vi "Func-Cp Cpk Calculation.vi"(0 "Uper limit":dbl=3.5, 5 "Lower limit":dbl=-3.5) -> (4 "Cp":dbl=1.932085875109604 format="%.3g", 6 "Cpk":dbl=1.7472929403358046 format="%.3g", 8 "Mean":dbl=-0.33475492991304356 format="%.3g", 10 "Variance":dbl=0.3646202027387419 format="%.3g", 15 "Standard deviation":dbl=0.6038378944209629 format="%.3g")   [LabVIEW 2015]
doc: "This Vi calculate the Cp and CPK of the population given by the Samples array.\nThe Upper and Lower limits need to be defined.\n\nCp= (UL-LL)/6*STD\n\nCpk= min((UL-MEAN)/3*STD,(MEAN-LL)/3*STD)"
panel:
  out "Data Length":dbl
  in  "문자열":string="-1.851121686\n-1.781249213\n-1.696262244\n-1.641406584\n-1.621321948\n-1.616843911\n-1.608642305\n-1.605459775\n-1.493903028\n-1.487135688\n-1.458574686\n-1.438584113\n-1.401760042\n-1.394260952\n-1.384378735\n-1.37466157\n-1.365849199\n-1.363884408\n-1.355128293\n-1.316161593\n-1.308444406\n-1.303143799\n-1.302773604\n-1.296959111\n-1.293790032\n-1.29178707\n-1.291699252\n-1.27635186\n-1.271757302\n-1.268175534\n-1.267821287\n-1.251471286\n-1.247559272\n-1.242962705\n-1.217645946\n-1.21736537\n-1.216009329\n-1.202190878\n-1.202112903\n-1.184886488\n-1.173962668\n-1.149552199\n-1.136492305\n-1.127663749\n-1.110186203\n-1.098839323\n-1.063263064\n-1.062590809\n-1.051174206\n-1.0350763\n-1.032616366\n-1.00586889\n-0.995767692\n-0.995159837\n-0.98525165\n-0.98196329\n-0.972898372\n-0.972202493\n-0.969240769\n-0.966011738\n-0.96122316\n-0.94254499\n-0.939456673\n-0.938051333\n-0.935893697\n-0.935341622\n-0.897347145\n-0.890632717\n-0.86677152\n-0.845623437\n-0.837863263\n-0.828699643\n-0.823162949\n-0.811628868\n-0.793890961\n-0.791592424\n-0.788485692\n-0.786059864\n-0.776439468\n-0.771175421\n-0.756713774\n-0.754180178\n-0.747972924\n-0.738974146\n-0.737735115\n-0.723125192\n-0.698505909\n-0.696495782\n-0.691014879\n-0.670102994\n-0.663213134\n-0.660173614\n-0.643176556\n-0.635550406\n-0.626554908\n-0.608300396\n-0.606095093\n-0.603400726\n-0.598510082\n-0.595354462\n-0.587561998\n-0.573913422\n-0.568345424\n-0.563687462\n-0.559160184\n-0.558902732\n-0.555301825\n-0.553530709\n-0.54605119\n-0.529988326\n-0.529235425\n-0.527026006\n-0.522869476\n-0.518973731\n-0.514763869\n-0.505587081\n-0.493579546\n-0.48985599\n-0.483537969\n-0.482482696\n-0.482414954\n-0.473320334\n-0.469467348\n-0.452348175\n-0.450832215\n-0.449496242\n-0.429675481\n-0.409118479\n-0.39707189\n-0.39029414\n-0.387083507\n-0.374743861\n-0.372941622\n-0.366007281\n-0.365920883\n-0.355394283\n-0.344413404\n-0.344094986\n-0.343650937\n-0.341575713\n-0.338731268\n-0.336521056\n-0.329717088\n-0.328186516\n-0.323740937\n-0.319114235\n-0.308047398\n-0.28295137\n-0.267773552\n-0.259518923\n-0.253211829\n-0.249036273\n-0.243012895\n-0.237937552\n-0.23472351\n-0.232765954\n-0.223881206\n-0.223762676\n-0.22323105\n-0.217884653\n-0.212155625\n-0.204602339\n-0.204030259\n-0.20356409\n-0.203086061\n-0.198433808\n-0.196635345\n-0.163945006\n-0.163916103\n-0.155360134\n-0.155235253\n-0.154121349\n-0.153919542\n-0.153388318\n-0.152636873\n-0.152481181\n-0.148134082\n-0.142589632\n-0.137008774\n-0.12647245\n-0.12557343\n-0.123881016\n-0.123868314\n-0.11561664\n-0.112112685\n-0.110043305\n-0.109985044\n-0.109723737\n-0.10594016\n-0.105639606\n-0.10355686\n-0.098659515\n-0.098607281\n-0.098373005\n-0.097118634\n-0.083297148\n-0.080455933\n-0.073766276\n-0.07251092\n-0.066247023\n-0.066247023\n-0.066045286\n-0.065259828\n-0.065034475\n-0.064515914\n-0.063829331\n-0.0599048\n-0.05223549\n-0.044948423\n-0.041152963\n-0.040847343\n-0.040683052\n-0.037970251\n-0.036130264\n-0.035842174\n-0.035620097\n-0.03546074\n-0.024837646\n-0.02259679\n-0.01924693\n-0.016197163\n-0.016091187\n-0.01588367\n-0.011912752\n-0.006533642\n-0.005783903\n-0.003741178\n-0.003713395\n-0.003698459\n-0.003577473\n0.006200636\n0.011377763\n0.015778103\n0.015778103\n0.016070206\n0.016334106\n0.028680123\n0.030356774\n0.03915029\n0.039653662\n0.05319111\n0.058159657\n0.059563761\n0.06034195\n0.060739363\n0.066268031\n0.067494866\n0.068603246\n0.06922644\n0.072871725\n0.07605783\n0.076936527\n0.079414977\n0.079762012\n0.081142904\n0.082046134\n0.083565072\n0.084937352\n0.08782068\n0.091087502\n0.099370535\n0.100358088\n0.108766379\n0.110649415\n0.137418853\n0.148535792\n0.16266193\n0.163330082\n0.169662436\n0.170493134\n0.222483436\n0.224152793\n0.230313209\n0.233322205\n0.234858871\n0.236222397\n0.237311582\n0.241024203\n0.258638946\n0.263582537\n0.282529822\n0.282695385\n0.286810418\n0.28940767\n0.296042548\n0.303273661\n0.304498374\n0.306697703\n0.306776635\n0.308335936\n0.323135697\n0.323585227\n0.330028997\n0.365758605\n0.386946878\n0.399114248\n0.409314606\n0.415204252\n0.431875391\n0.444799699\n0.466200899\n0.487349548\n0.491379186\n0.534357688\n0.536321157\n0.552104532\n0.553079385\n0.583193698\n0.600169278\n0.720360649\n0.722727719\n0.773414334\n0.827668935\n0.861770406\n0.868698608\n0.90552577\n1.02005817\n1.108558767\n1.130760164\n1.154642797\n1.223375919\n1.273115061"
  out "Samples":dbl[](array[numeric])=[-1.851121686, -1.781249213, -1.696262244, -1.641406584, -1.621321948, -1.616843911, -1.608642305, -1.605459775, -1.493903028, -1.487135688, -1.458574686, -1.438584113, -1.401760042, -1.394260952, -1.384378735, -1.37466157, -1.365849199, -1.363884408, -1.355128293, -1.316161593, -1.308444406, -1.303143799, -1.302773604, -1.296959111, -1.293790032, -1.29178707, -1.291699252, -1.27635186, -1.271757302, -1.268175534, -1.267821287, -1.251471286, -1.247559272, -1.242962705, -1.217645946, -1.21736537, -1.216009329, -1.202190878, -1.202112903, -1.184886488, -1.173962668, -1.149552199, -1.136492305, -1.127663749, -1.110186203, -1.098839323, -1.063263064, -1.062590809, -1.051174206, -1.0350763, -1.032616366, -1.00586889, -0.995767692, -0.995159837, -0.98525165, -0.98196329, -0.972898372, -0.972202493, -0.969240769, -0.966011738, -0.96122316, -0.94254499, -0.939456673, -0.938051333, -0.935893697, -0.935341622, -0.897347145, -0.890632717, -0.86677152, -0.845623437, -0.837863263, -0.828699643, -0.823162949, -0.811628868, -0.793890961, -0.791592424, -0.788485692, -0.786059864, -0.776439468, -0.771175421, -0.756713774, -0.754180178, -0.747972924, -0.738974146, -0.737735115, -0.723125192, -0.698505909, -0.696495782, -0.691014879, -0.670102994, -0.663213134, -0.660173614, -0.643176556, -0.635550406, -0.626554908, -0.608300396, -0.606095093, -0.603400726, -0.598510082, -0.595354462, -0.587561998, -0.573913422, -0.568345424, -0.563687462, -0.559160184, -0.558902732, -0.555301825, -0.553530709, -0.54605119, -0.529988326, -0.529235425, -0.527026006, -0.522869476, -0.518973731, -0.514763869, -0.505587081, -0.493579546, -0.48985599, -0.483537969, -0.482482696, -0.482414954, -0.473320334, -0.469467348, -0.452348175, -0.450832215, -0.449496242, -0.429675481, -0.409118479, -0.39707189, -0.39029414, -0.387083507, -0.374743861, -0.372941622, -0.366007281, -0.365920883, -0.355394283, -0.344413404, -0.344094986, -0.343650937, -0.341575713, -0.338731268, -0.336521056, -0.329717088, -0.328186516, -0.323740937, -0.319114235, -0.308047398, -0.28295137, -0.267773552, -0.259518923, -0.253211829, -0.249036273, -0.243012895, -0.237937552, -0.23472351, -0.232765954, -0.223881206, -0.223762676, -0.22323105, -0.217884653, -0.212155625, -0.204602339, -0.204030259, -0.20356409, -0.203086061, -0.198433808, -0.196635345, -0.163945006, -0.163916103, -0.155360134, -0.155235253, -0.154121349, -0.153919542, -0.153388318, -0.152636873, -0.152481181, -0.148134082, -0.142589632, -0.137008774, -0.12647245, -0.12557343, -0.123881016, -0.123868314, -0.11561664, -0.112112685, -0.110043305, -0.109985044, -0.109723737, -0.10594016, -0.105639606, -0.10355686, -0.098659515, -0.098607281, -0.098373005, -0.097118634, -0.083297148, -0.080455933, -0.073766276, -0.07251092, -0.066247023, -0.066247023, -0.066045286, -0.065259828, -0.065034475, -0.064515914, -0.063829331, -0.0599048, -0.05223549, -0.044948423, -0.041152963, -0.040847343, -0.040683052, -0.037970251, -0.036130264, -0.035842174, -0.035620097, -0.03546074, -0.024837646, -0.02259679, -0.01924693, -0.016197163, -0.016091187, -0.01588367, -0.011912752, -0.006533642, -0.005783903, -0.003741178, -0.003713395, -0.003698459, -0.003577473, 0.006200636, 0.011377763, 0.015778103, 0.015778103, 0.016070206, 0.016334106, 0.028680123, 0.030356774, 0.03915029, 0.039653662, 0.05319111, 0.058159657, 0.059563761, 0.06034195, 0.060739363, 0.066268031, 0.067494866, 0.068603246, 0.06922644, 0.072871725, 0.07605783, 0.076936527, 0.079414977, 0.079762012, 0.081142904, 0.082046134, 0.083565072, 0.084937352, 0.08782068, 0.091087502, 0.099370535, 0.100358088, 0.108766379, 0.110649415, 0.137418853, 0.148535792, 0.16266193, 0.163330082, 0.169662436, 0.170493134, 0.222483436, 0.224152793, 0.230313209, 0.233322205, 0.234858871, 0.236222397, 0.237311582, 0.241024203, 0.258638946, 0.263582537, 0.282529822, 0.282695385, 0.286810418, 0.28940767, 0.296042548, 0.303273661, 0.304498374, 0.306697703, 0.306776635, 0.308335936, 0.323135697, 0.323585227, 0.330028997, 0.365758605, 0.386946878, 0.399114248, 0.409314606, 0.415204252, 0.431875391, 0.444799699, 0.466200899, 0.487349548, 0.491379186, 0.534357688, 0.536321157, 0.552104532, 0.553079385, 0.583193698, 0.600169278, 0.720360649, 0.722727719, 0.773414334, 0.827668935, 0.861770406, 0.868698608, 0.90552577, 1.02005817, 1.108558767, 1.130760164, 1.154642797, 1.223375919, 1.273115061] format="%0.2f"
  # "공정능력분석(Cp,Cpk,Pp,Ppk)"
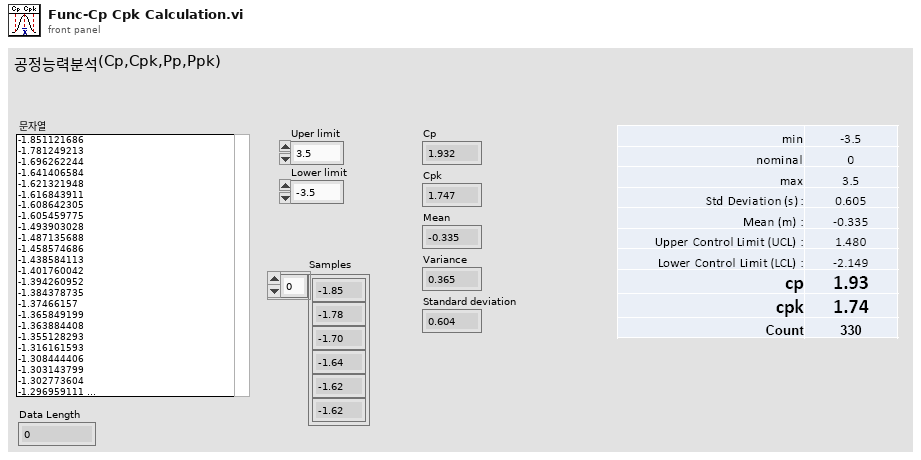
[diagram p1: front panel]
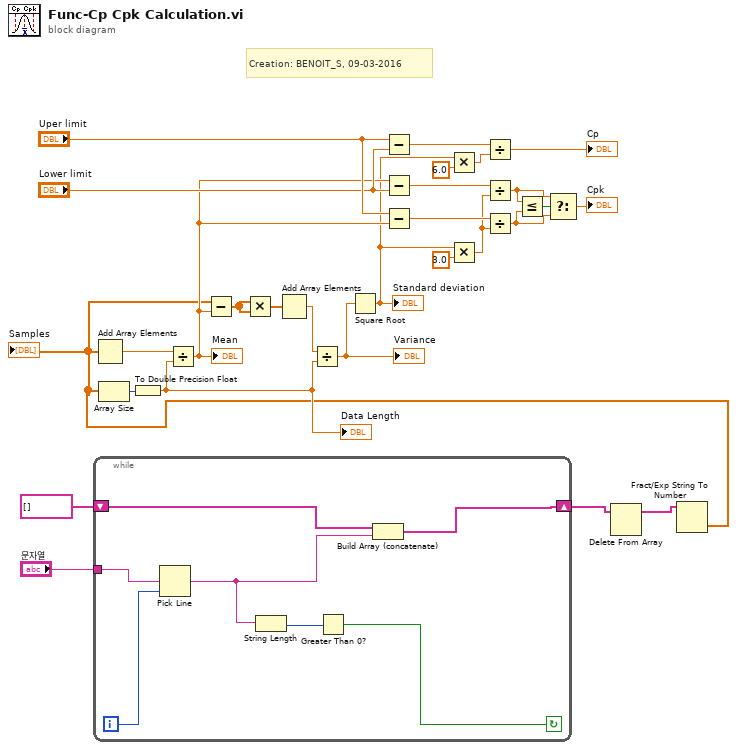
[diagram p0: block diagram]
diagram:
  # "Creation: BENOIT_S, 09-03-2016"
  n1 = while {
    tunnel: "문자열" -> [w35]
    shift-right: [w33] -> w3
    shift-left: string[] [] -> [w34]
    i -> [w32]
    stop <- w29 continue-if-true
    n2 = Pick Line(multi-line string=w35, line index=w32) -> (output string=w31:string)  [unwired: 1 in]
    n3 = String Length(string=w31) -> (length=w30:i32)
    n4 = Greater Than 0?(x=w30) -> (x > 0?=w29:bool)
    n5 = Build Array (concatenate)(w34, w31) -> (w33:string[])
  }
  n6 = Subtract(x="Uper limit", y="Lower limit") -> (x-y=w28:dbl)
  n7 = Delete From Array(array=w3) -> (array with subset deleted=w2:string[])  [unwired: 2 in, 1 out]
  n8 = Fract/Exp String To Number(string=w2) -> (number=w1:dbl[])  [unwired: 3 in, 1 out]
  "Samples" <- w1
  n9 = Add Array Elements(numeric array=w1) -> (sum=w13:dbl)
  n10 = Array Size(array=w1) -> (size(s)=w14:i32)
  n11 = To Double Precision Float(number=w14) -> (double precision float=w9:dbl)
  "Data Length" <- w9
  n12 = Divide(x=w13, y=w9) -> (x/y=w7:dbl)
  "Mean" <- w7
  n13 = Subtract(x=w1, y=w7) -> (x-y=w12:dbl[])
  n14 = Multiply(x=w12, y=w12) -> (x*y=w11:dbl[])
  n15 = Add Array Elements(numeric array=w11) -> (sum=w10:dbl)
  n16 = Divide(x=w10, y=w9) -> (x/y=w8:dbl)
  "Variance" <- w8
  n17 = Square Root(x=w8) -> (sqrt(x)=w6:dbl)
  "Standard deviation" <- w6
  n18 = Subtract(x=w7, y="Lower limit") -> (x-y=w23:dbl)
  n19 = Subtract(x="Uper limit", y=w7) -> (x-y=w22:dbl)
  n20 = Multiply(x=w6, y=6.0 ("x")) -> (x*y=w27:dbl)
  n21 = Multiply(x=w6, y=3.0 ("x")) -> (x*y=w21:dbl)
  n22 = Divide(x=w28, y=w27) -> (x/y=→"Cp":dbl)
  n23 = Divide(x=w23, y=w21) -> (x/y=w18:dbl)
  n24 = Divide(x=w22, y=w21) -> (x/y=w17:dbl)
  n25 = Less Or Equal?(x=w18, y=w17) -> (x <= y?=w19:bool)
  n26 = Select(t=w18, s=w19, f=w17) -> (s? t:f=→"Cpk":dbl)
